vi "SUBVI_step_fn_raman.vi"(9 "i":dbl, 10 "Step Size / [µm]":dbl, 11 "Move / [µm]":dbl) -> (2 "y / [µm]":dbl, 3 "x / [µm]":dbl, 5 "done?":bool)   [LabVIEW 2020]
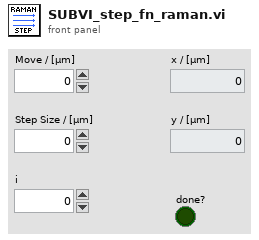
[diagram p1: front panel]
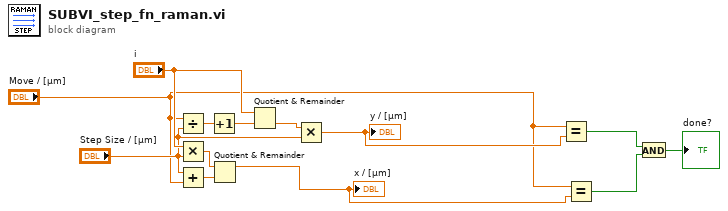
[diagram p0: block diagram]
diagram:
  n1 = Divide(x="Move / [µm]", y="Step Size / [µm]") -> (x/y=w13:dbl)
  n2 = Multiply(x="i", y="Step Size / [µm]") -> (x*y=w8:dbl)
  n3 = Add(x="Step Size / [µm]", y="Move / [µm]") -> (x+y=w7:dbl)
  n4 = Increment(x=w13) -> (x+1=w11:dbl)
  n5 = Quotient & Remainder(x=w8, y=w7) -> (x-y*floor(x/y)=w4:dbl)  [unwired: 1 out]
  "x / [µm]" <- w4
  n6 = Quotient & Remainder(x="i", y=w11) -> (floor(x/y)=w10:dbl)  [unwired: 1 out]
  n7 = Multiply(x=w10, y="Step Size / [µm]") -> (x*y=w6:dbl)
  "y / [µm]" <- w6
  n8 = Equal?(x="Move / [µm]", y=w6) -> (x = y?=w3:bool)
  n9 = Equal?(x="Move / [µm]", y=w4) -> (x = y?=w2:bool)
  n10 = And(x=w3, y=w2) -> (x .and. y?=→"done?":bool)
